vi "Mode_read.vi"(4 "error in (no error)":errorcluster, 6 "Container State":T2, 7 "Display State In":T1 {"Mode" items=["U DC", "U AC", "I DC", "I AC", "R"]}) -> (0 "error out":errorcluster, 2 "Value":u8, 3 "Display State Out":T1 {"Mode" items=["U DC", "U AC", "I DC", "I AC", "R"]})   [LabVIEW 2020, in "Multimetr.xctl"]
uses:
  Multimetr.xctl
  <vilib>/_xctls/Container State.ctl
  Multimetr-state.ctl
  <vilib>/_xctls/XControlSupport.lvlib
panel:
  # "Replace the Value Indicator below with an Indicator of desired type.\nDo not remove this Indicator or the others from the connector pane. \nDo not change the connector pane pattern.\nThe Value Indicator should always be the second terminal from top on the output side in the connector pane."
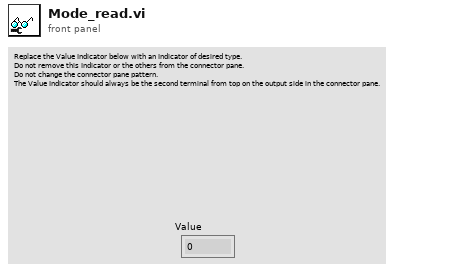
[diagram p1: front panel]
types:
  T1 = typedef "Multimetr.xctl/Multimetr-state.ctl" = cluster{"ON":bool, "Mode":u16, "I connected?":bool, "U connected?":bool}
  T2 = typedef "XControlSupport.lvlib/Container State.ctl" = cluster{"Indicator?":bool, "Run Mode?":bool, " Refnum":refnum<vi>}
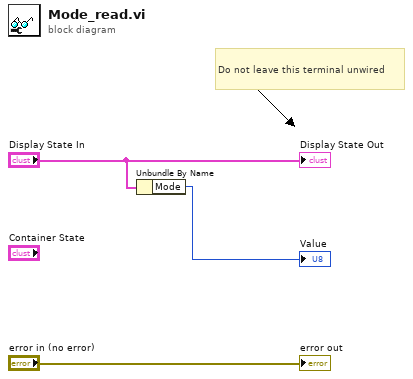
[diagram p0: block diagram]
diagram:
  # "Do not leave this terminal unwired"
  n1 = Unbundle By Name("Display State In") -> ("Mode"=→"Value":u16)
  "error out" <- "error in (no error)"
  "Display State Out" <- "Display State In"
